vi "16TVTI-WriteAutoMode.vi"(1 "Auto Needle Valve":bool, 2 "Auto Heat":bool, 3 "Instrument address":T1) -> (0 "Instrument address (out)":T1)   [LabVIEW 2019]
doc: "Sets the control modes of the ITC."
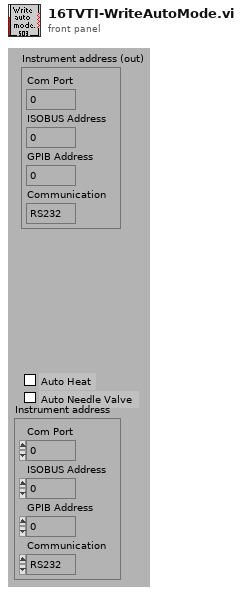
[diagram p1: front panel]
types:
  T1 = cluster{"Com Port":i32, "ISOBUS Address":i32, "GPIB Address":i16, "Communication":enum16{"RS232", "ISOBUS", "GPIB", "Gateway"}}
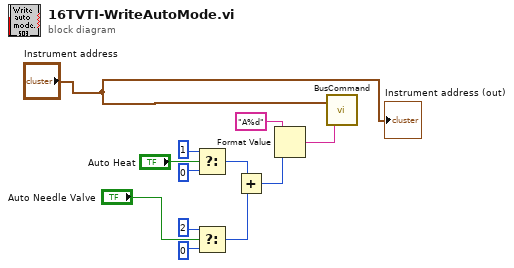
[diagram p0: block diagram]
diagram:
  n1 = Select(t=1, s="Auto Heat", f=0) -> (s? t:f=w6:i32)
  n2 = Select(t=2, s="Auto Needle Valve", f=0) -> (s? t:f=w5:i32)
  n3 = Add(x=w6, y=w5) -> (x+y=w4:i32)
  n4 = Format Value(format string="A%d", value (0)=w4) -> (output string=w12:string)  [unwired: 1 in]
  n5 = call "BusCommand.vi"("Command"=w12, "Instrument address (in)"="Instrument address") -> ()  [unwired: 2 out]
  "Instrument address (out)" <- "Instrument address"
